vi "ECT in Standby State.vi"(0 "GEA2 Reference In":refnum<k24>, 5 "Option Selection":T2={"Soil Level"=enum."Normal", "Warm Rinse"=enum."Disable", "Fabric Softener"=enum."Disable", "Extra Rinse"=enum."Disable", "Soak"=enum."Level 0", "Stain"=enum."Off", "Spin"=enum."Normal Spin", "Load Size"=enum."Precise Fill", "Dry Load Size"=enum."65535", "Load Type"=enum."Unknown", "Deep Fill"=enum."Off"}, 7 "ECT Parameters":T1={"MS to Spin Time"=0, "Target Fill Time"=238, "MS to Agitate Time"=0, "MS to Spin before Spin Time "=0, "Adaptive Drain Time"=180, "Coast to 0 Time"=60}, 11 "Error In":errorcluster) -> (3 "Expected SSD in Standby":string, 4 "GEA2 Reference Out":refnum<k24>, 6 "Expected ECT in Standby (sec)":u16, 8 "Actual ECT in Standby (sec)":u16, 10 "ECT Standby Pass/Fail":bool, 14 "Report Text in Standby":string, 15 "Error Out":errorcluster)   [LabVIEW 2016, in "Centauro.lvlib"]
doc: "This vi can be used to read ERD every 1 sec for user selected repeat counts."
uses:
  Projects/Centauro.lvlib
  Common/LabVIEW GEA2 Toolkit/LabVIEW_GEA2_Toolkit.lvlibp
  Valew Common/type defs/Encoder Position.ctl
  Common/LabVIEW GEA2 Toolkit/LabVIEW_GEA2_Toolkit.lvlibp/type defs/ERD Write Data In.ctl
  Common/LabVIEW GEA2 Toolkit/LabVIEW_GEA2_Toolkit.lvlibp/type defs/Source_Destination.ctl
  Common/LabVIEW GEA2 Toolkit/LabVIEW_GEA2_Toolkit.lvlibp/type defs/Data Type.ctl
  Q:/Common/DLLs/GEA3/GeaCommunication.dll
  Common/DLLs/GEA3/GeaCommunication.dll
  Controls/Options.ctl
  Controls/ECT Parameters.ctl
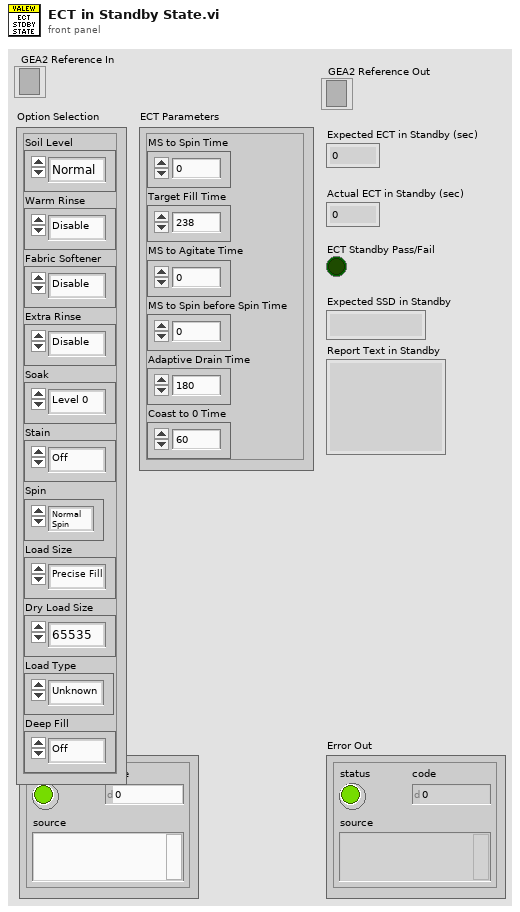
[diagram p1: front panel]
types:
  T1 = typedef "Centauro.lvlib/ECT Parameters.ctl" = cluster{"MS to Spin Time":u16, "Target Fill Time":u16, "MS to Agitate Time":u16, "MS to Spin before Spin Time ":u16, "Adaptive Drain Time":u16, "Coast to 0 Time":u16}
  T2 = typedef "Centauro.lvlib/Options.ctl" = cluster{"Soil Level":enum8{"Ex Light", "Light", "Normal", "Heavy", "Ex Heavy"}, "Warm Rinse":enum8{"Disable", "Enable"}, "Fabric Softener":enum16{"Disable", "Enable"}, "Extra Rinse":enum8{"Disable", "Enable"}, "Soak":enum8{"Level 0", "Level 1", "Level 2", "Level 3", "Level 4"}, "Stain":enum8{"Off", "Tomato", "Wine", "Blood", "Grass", "Dirt"}, "Spin":enum16{"No Spin", "Normal Spin", "More Spin", "Max Spin"}, "Load Size":enum8{"Small", "Medium", "Large", "Super", "Precise Fill", "Super Plus"}, "Dry Load Size":enum16{"128", "256", "384", "5AA", "6A4", "834", "65535"}, "Load Type":enum8{"Unknown", "Cotton", "Synthetic", "Mixed", "Wet", "Low Flow", "Small", "Medium", "Large", "Super", "Super Plus", "Max"}, "Deep Fill":enum8{"Off", "Incremental Fill", "Max Fill"}}
  T3 = typedef "LabVIEW_GEA2_Toolkit.lvlibp/Source_Destination.ctl" = cluster{"Source":u8, "Destination":u8}
  T4 = typedef "LabVIEW_GEA2_Toolkit.lvlibp/ERD Write Data In.ctl" = cluster{"ERD Number":u16, "Data Type":T5, "Data":string}
  T5 = typedef "LabVIEW_GEA2_Toolkit.lvlibp/Data Type.ctl" = enum16{"string", "boolean", "uint8_t", "uint16_t", "uint32_t", "uint64_t", "int8_t", "int16_t", "int32_t", "int64_t"}
  T6 = typedef "Centauro.lvlib/Encoder Position.ctl" = enum16{"Position 0", "Position 1", "Position 2", "Position 3", "Position 4", "Position 5", "Position 6", "Position 7", "Position 8", "Position 9", "Position 10", "Position 11", "Position 12", "Position 13", "Clear / Reset"}
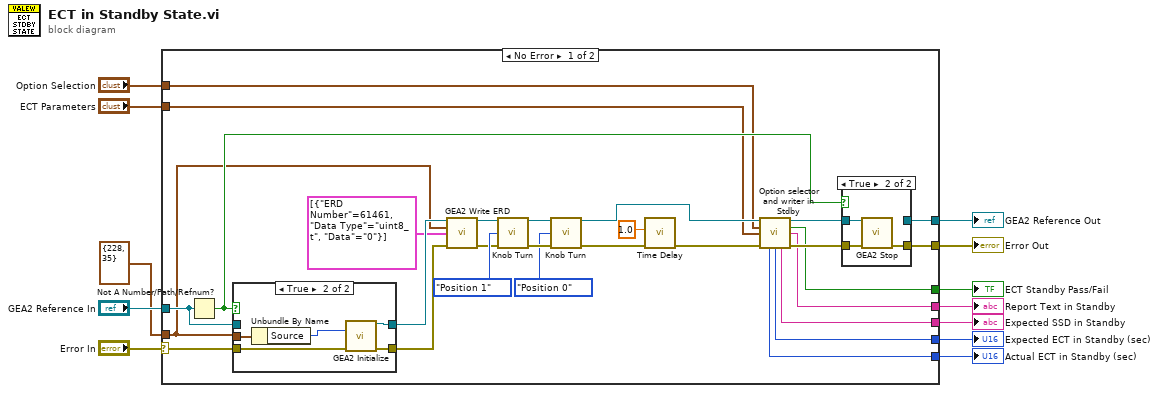
[diagram p0: block diagram]
diagram:
  n1 = case shown="No Error" "Error In" {
    selector: "Error In" -> [w39 w53]
    tunnel: T3 {"Source"=228, "Destination"=35} ("GEA Inputs") -> [w23 _]
    tunnel: "GEA2 Reference In" -> [w40 w54]
    tunnel: [w25 w54] -> w10
    tunnel: [w27 w53] -> w9
    tunnel: "Option Selection" -> [w14 _]
    tunnel: [w19 _] -> w6
    tunnel: [w18 _] -> w5
    tunnel: [w17 _] -> w4
    tunnel: [w16 _] -> w3
    tunnel: [w15 _] -> w2
    tunnel: "ECT Parameters" -> [w13 _]
    frame No Error {
      n2 = Not A Number/Path/Refnum?(number/path/refnum=w40) -> (NaN/Path/Refnum?=w29:bool)
      n3 = case shown="True" w29 {
        tunnel: w39 -> [w47 w52]
        tunnel: [w47 w51] -> w34
        tunnel: [w46 w50] -> w33
        tunnel: w23 -> [_ w48]
        tunnel: w40 -> [w46 _]
        frame False {
        }
        frame True {
          n4 = Unbundle By Name(w48) -> ("Source"=w49:u8)
          n5 = call "GEA2 Initialize.vi"("Source Address"=w49, "error in"=w52) -> ("GEA2 Reference Out"=w50:refnum<k24>, "error out"=w51:errorcluster)  [unwired: 11 in, 1 out]
        }
      }
      n6 = call "GEA2 Write ERD.vi"("GEA2 Reference In"=w33, "GEA Inputs"=w23, "Write ERD List"=T4[] [{"ERD Number"=61461, "Data Type"=enum."uint8_t", "Data"="0"}], "Error In"=w34) -> ("GEA2 Reference Out"=w32:refnum<k24>, "Error Out"=w31:errorcluster)  [unwired: 9 in, 1 out]
      n7 = call "Knob Turn.vi"("GEA2 Reference In"=w32, "Button"=Encoder_Position."Position 1", "Error In"=w31) -> ("GEA2 Reference Out"=w37:refnum<k24>, "Error Out"=w36:errorcluster)  [unwired: 11 in]
      n8 = call "Knob Turn.vi"("GEA2 Reference In"=w37, "Button"=Encoder_Position."Position 0", "Error In"=w36) -> ("GEA2 Reference Out"=w28:refnum<k24>, "Error Out"=w24:errorcluster)  [unwired: 11 in]
      n9 = call "Time Delay"("error in (no error)"=w24, "Delay Time (s)"=1.0) -> ("error out"=w22:errorcluster)  [unwired: 9 in]
      n10 = call "Option selector and writer in Stdby.vi"(".NET Refnum in"=w28, "Option Selection"=w14, "ECT Parameters"=w13, "error in (no error)"=w22) -> (".NET Refnum out"=w26:refnum<k24>, "ECT Pass/Fail"=w19:bool, "Report Text"=w18:string, "Actual ECT (sec)"=w15:u16, "Expected ECT (sec)"=w16:u16, "Expected SSD"=w17:string, "error out"=w21:errorcluster)  [unwired: 5 in]
      n11 = case shown="True" w29 {
        tunnel: [w41 w45] -> w27
        tunnel: w26 -> [w42 w44]
        tunnel: [w42 _] -> w25
        tunnel: w21 -> [w41 w43]
        frame False {
        }
        frame True {
          n12 = call "GEA2 Stop.vi"("GEA2 Reference In"=w44, "Error In"=w43) -> ("Error Out"=w45:errorcluster)  [unwired: 13 in]
        }
      }
    }
    frame Error {
    }
  }
  "GEA2 Reference Out" <- w10
  "Error Out" <- w9
  "Expected SSD in Standby" <- w4
  "Expected ECT in Standby (sec)" <- w3
  "Actual ECT in Standby (sec)" <- w2
  "ECT Standby Pass/Fail" <- w6
  "Report Text in Standby" <- w5
